vi "Write Additional Labels to File.vi"(8 "error in (no error)":errorcluster, 11 "Control Info in":refnum<class "Control Info.lvclass">) -> (0 "error out":errorcluster, 3 "Control Info out":refnum<class "Control Info.lvclass">)   [LabVIEW 2017, in "Localization.lvlib" / "Control Info.lvclass"]
doc: "Writes all of the Alternate Text label information to the INI file for the specified Control.\n\nChoose Movement Consulting, LLC"
uses:
  Control Info.lvclass
  Control Info.lvclass/Control Info.ctl
  <vilib>/Utility/NIReport.llb/Append Text Table to Report (wrap).vi
  <vilib>/Utility/NIReport.llb/NI_report.lvclass
  <vilib>/Utility/NIReport.llb/Excel/NI_Excel.lvclass
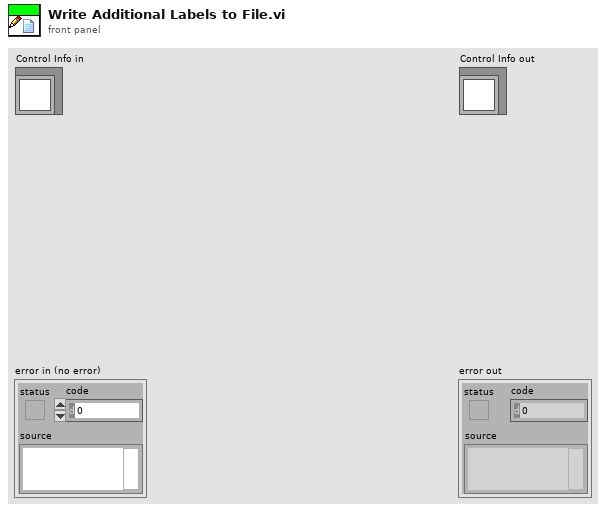
[diagram p1: front panel]
types:
  T1 = enum16{"Standard Report", "HTML", "Word", "Excel"}
  T2 = cluster{"on/off":bool, "weight":i32, "color":u32}
  T3 = cluster{"position (excel)":cluster{"row":i32, "column":i32}, "name (excel)":string, "bookmark (word)":string}
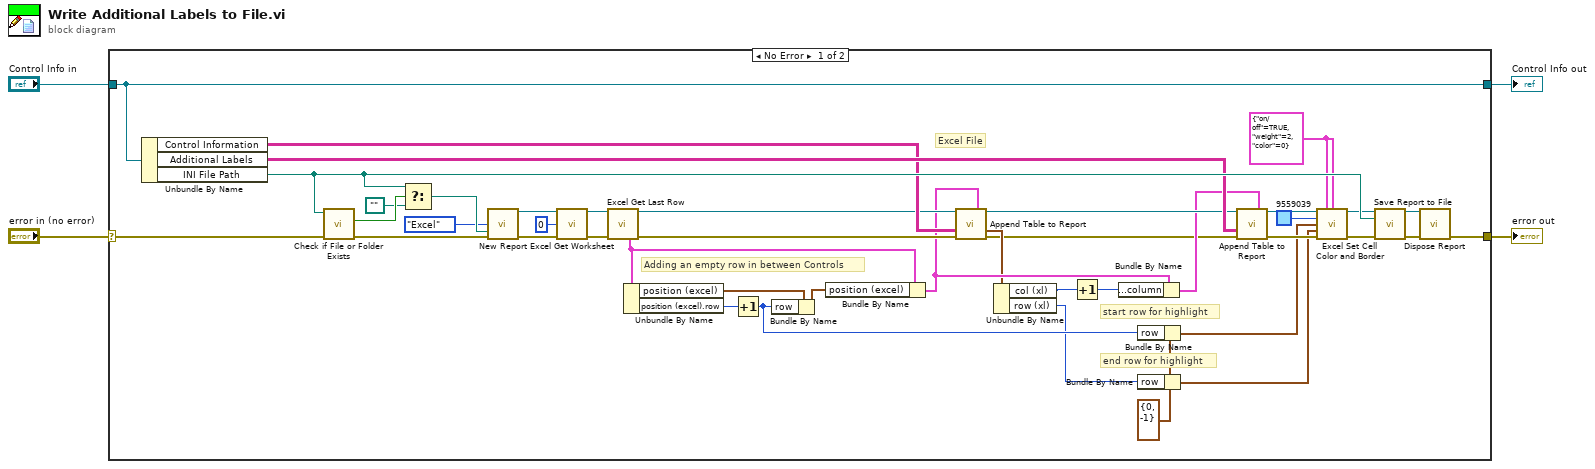
[diagram p0: block diagram]
diagram:
  n1 = case shown="No Error" "error in (no error)" {
    selector: "error in (no error)" -> [w45 w48]
    tunnel: [w43 w48] -> w3
    tunnel: [w44 w47] -> w1
    tunnel: "Control Info in" -> [w44 w47]
    frame No Error {
      w6 = T2 {"on/off"=TRUE, "weight"=2, "color"=0} ("outside border")
      w20 = cluster{"row":i32, "column":i32} {"row"=0, "column"=-1} ("position (excel)")
      # "end row for highlight"
      # "start row for highlight"
      # "Adding an empty row in between Controls"
      # "Excel File"
      n2 = Unbundle By Name(w44) -> ("Control Information"=w41:string[][], "Additional Labels"=w42:string[][], "INI File Path"=w46:path)
      n3 = call <vilib>:"Check if File or Folder Exists.vi"("error in (no error)"=w45, "path"=w46) -> ("error out"=w10:errorcluster, "file or folder exists?"=w9:bool)  [unwired: 7 in, 1 out]
      n4 = Select(t=w46, s=w9, f=path "" ("template (empty)")) -> (s? t:f=w7:path)
      n5 = call <vilib>:"New Report.vi"("report type"=T1."Excel", "template (empty)"=w7, "error in (no error)"=w10) -> ("report out"=w37:refnum<class "NI_report.lvclass">, "error out"=w38:errorcluster)  [unwired: 11 in]
      n6 = call <vilib>:"Excel Get Worksheet.vi"("report in"=w37, "worksheet index (0)"=0, "error in (no error)"=w38) -> ("report out"=w39:refnum<class "NI_report.lvclass">, "error out"=w40:errorcluster)  [unwired: 11 in]
      n7 = call <vilib>:"Excel Get Last Row.vi"("report in"=w39, "error in (no error)"=w40) -> ("report out"=w36:refnum<class "NI_report.lvclass">, "MS Office parameters out"=w31:T3, "error out"=w35:errorcluster)  [unwired: 11 in]
      n8 = Unbundle By Name(w31) -> ("position (excel)"=w33:cluster{"row":i32, "column":i32}, "position (excel).row"=w32:i32)
      n9 = Increment(x=w32) -> (x+1=w29:i32)
      n10 = Bundle By Name(cluster=w33, "row"=w29) -> (w30:cluster{"row":i32, "column":i32})
      n11 = Bundle By Name(cluster=w31, "position (excel)"=w30) -> (w27:T3)
      n12 = call-poly <vilib>:"Append Table to Report.vi"("report in"=w36, "MS Office parameters"=w27, "text data"=w41, "error in (no error)"=w35) -> ("report out"=w28:refnum<class "NI_report.lvclass">, "end (xl)"=w26:cluster{"row (xl) ":i32, "col (xl) ":i32}, "error out"=w22:errorcluster)  [unwired: 8 in, 1 out]
      n13 = Unbundle By Name(w26) -> ("col (xl)"=w25:i32, "row (xl)"=w21:i32)
      n14 = Increment(x=w25) -> (x+1=w24:i32)
      n15 = Bundle By Name(cluster=w27, "position (excel).column"=w24) -> (w23:T3)
      n16 = Bundle By Name(cluster=w20, "row"=w29) -> (w16:cluster{"row":i32, "column":i32})
      n17 = Bundle By Name(cluster=w20, "row"=w21) -> (w15:cluster{"row":i32, "column":i32})
      n18 = call-poly <vilib>:"Append Table to Report.vi"("report in"=w28, "MS Office parameters"=w23, "text data"=w42, "error in (no error)"=w22) -> ("report out"=w19:refnum<class "NI_report.lvclass">, "error out"=w18:errorcluster)  [unwired: 8 in, 2 out]
      n19 = call <vilib>:"Excel Set Cell Color and Border.vi"("report in"=w19, "inside border"=w6, "outside border"=w6, "background color (w)"=u32 9559039, "start (-1, -1)"=w16, "end (-1, -1)"=w15, "error in (no error)"=w18) -> ("report out"=w14:refnum<class "NI_report.lvclass">, "error out"=w13:errorcluster)  [unwired: 7 in]
      n20 = call-dynamic "Save Report to File.vi"("report in"=w14, "report file path"=w46, "error in (no error)"=w13) -> ("report out"=w11:refnum<class "NI_report.lvclass">, "error out"=w12:errorcluster)  [unwired: 11 in]
      n21 = call-dynamic "Dispose Report.vi"("report in"=w11, "error in (no error)"=w12) -> ("error out"=w43:errorcluster)  [unwired: 13 in]
    }
    frame Error {
    }
  }
  "error out" <- w3
  "Control Info out" <- w1
